vi "Write Data Bus.vi"(8 "error in (no error)":errorcluster, 10 "Data":u8 format="%02x", 11 "IO in":refnum<class "IO.lvclass">) -> (0 "error out":errorcluster)   [LabVIEW 2021, in "IO.lvclass"]
uses:
  IO.lvclass
  IO.lvclass/IO.ctl
  <vilib>/DAQmx/write.llb/DAQmx Write (Digital 1D Bool NChan 1Samp 1Line).vi
  <vilib>/DAQmx/miscellaneous.llb/DAQmx Fill In Error Info.vi
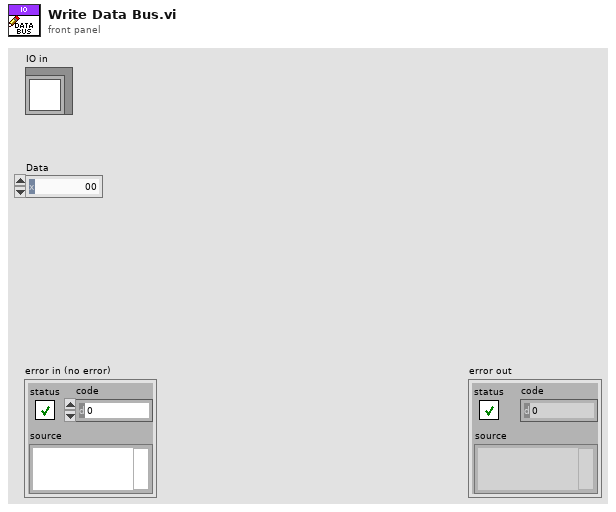
[diagram p1: front panel]
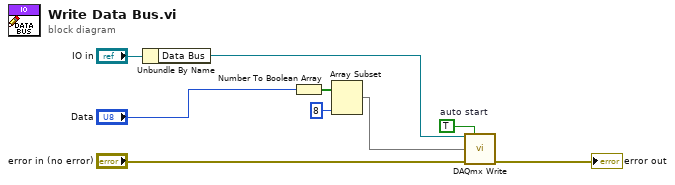
[diagram p0: block diagram]
diagram:
  w8 = TRUE  # auto start
  n1 = Unbundle By Name("IO in") -> ("Data Bus"=w3:refnum<k21>)
  n2 = Number To Boolean Array(number="Data") -> (Boolean array=w5:bool[])
  n3 = Array Subset(array=w5, length=8) -> (w1:bool[])  [unwired: 1 in]
  n4 = call-poly <vilib>:"DAQmx Write.vi"("task/channels in"=w3, "auto start"=w8, "data"=w1, "error in"="error in (no error)") -> ("error out"=→"error out":errorcluster)  [unwired: 9 in, 2 out]
